vi "Cam Heapsort.vi"(1 "Array":T1[](array[typedef])) -> (0 "Sorted Array":T1[](array[typedef]))   [LabVIEW 2018]
uses:
  Shared/Graham Scan/Graham Scan Point.ctl
  89644e54-da80-45d4-b50a-5ecc0376de4e.vi
  552978ab-fa66-4bb7-a624-dab1e7af6aa8.vi
  5754ab37-9295-44a8-8a21-49feac43d5eb.vi
  9c49b0bc-1d81-4ffb-947e-b2c48764fe7c.vi
  89644e54-da80-45d4-b50a-5ecc0376de4e.vi/2b2145cf-1d66-44f7-911e-bb5b6b170b9f.vi
  5754ab37-9295-44a8-8a21-49feac43d5eb.vi/c5ebe4f1-673c-4488-b403-7342dbc268ef.vi
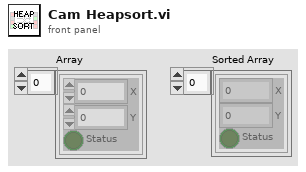
[diagram p1: front panel]
types:
  T1 = typedef "Graham Scan Point.ctl" = cluster{"X":i32, "Y":i32, "Status":bool}
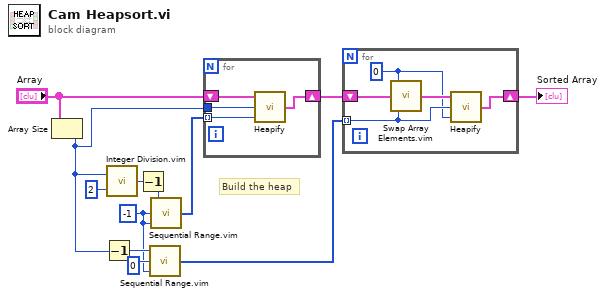
[diagram p0: block diagram]
diagram:
  w5 = -1 ("Stop")
  # "Build the heap"
  n1 = Array Size(array="Array") -> (size(s)=w1:i32)
  n2 = Decrement(x=w1) -> (x-1=w7:i32)
  n3 = call "Integer Division.vim"("Y"=2, "X"=w1) -> ("X // Y"=w10:i32)
  n4 = Decrement(x=w10) -> (x-1=w9:i32)
  n5 = call "Sequential Range.vim"("Increment (1)"=w5, "Stop"=0, "Start (0)"=w7) -> ("Range(st, stp, inc)"=w3:i32[])
  n6 = call "Sequential Range.vim"("Increment (1)"=w5, "Stop"=w5, "Start (0)"=w9) -> ("Range(st, stp, inc)"=w8:i32[])
  n7 = for {
    shift-right: [w15] -> w4
    shift-left: "Array" -> [w16]
    tunnel: w8 -> [w14] mode=indexing
    tunnel: w1 -> [w13]
    n8 = call "Heapify.vi"("Index"=w14, "Length"=w13, "Array"=w16) -> ("Heapified Array"=w15:T1[])
  }
  n9 = for {
    shift-right: [w17] -> w2
    shift-left: w4 -> [w21]
    tunnel: w3 -> [w19] mode=indexing
    w18 = 0 ("Index A")
    n10 = call "Swap Array Elements.vim"("Index B"=w19, "Array"=w21, "Index A"=w18) -> ("Array Out"=w20:T1[])
    n11 = call "Heapify.vi"("Index"=w18, "Length"=w19, "Array"=w20) -> ("Heapified Array"=w17:T1[])
  }
  "Sorted Array" <- w2
